vi "ScanBoxA.vi"(11 "YTESTER测试数据":T1 caption="不要修改！") -> (3 "YTESTER结论":T2)   [LabVIEW 2017]
doc: "VIDescription=异步调用一个扫码框！"
uses:
  YtCommon.lvlibp/yt`Step StepBaseInput.ctl
  YtCommon.lvlibp/yt`Step StepResult.ctl
  YtCommon.lvlibp/yt`Step TestData.ctl
  YtCommon.lvlibp/yt`Step System Queue.ctl
  74c99672-6dce-4f91-812f-8692ad59771d.vi
  <vilib>/Utility/error.llb/Clear Errors.vi
  YtCommon.lvlibp/yt`varSystemlib IO Read Variable.vi
  YtCommon.lvlibp
panel:
  in  "YTESTER开放参数":T4={"YTESTER_BaseInput"={"isTest"=FALSE, "isSkip"=FALSE, "StepName"="异步·扫码框A", "OnPass"=enum."Next", "OnFail"=enum."Next", "ReTestNumber"=0.0}, "扫码项目"=["SN："], "扫码项长度"=[], "扫码项文本头匹配"=[], "码不可重复"=TRUE, "窗口位置Left(100)"=100, "窗口位置Top(100)"=100, "满足全部扫码项目后延迟触发测试(s)慎用！"=-1.0, "触发哪些DUTs自动测试？"=""}
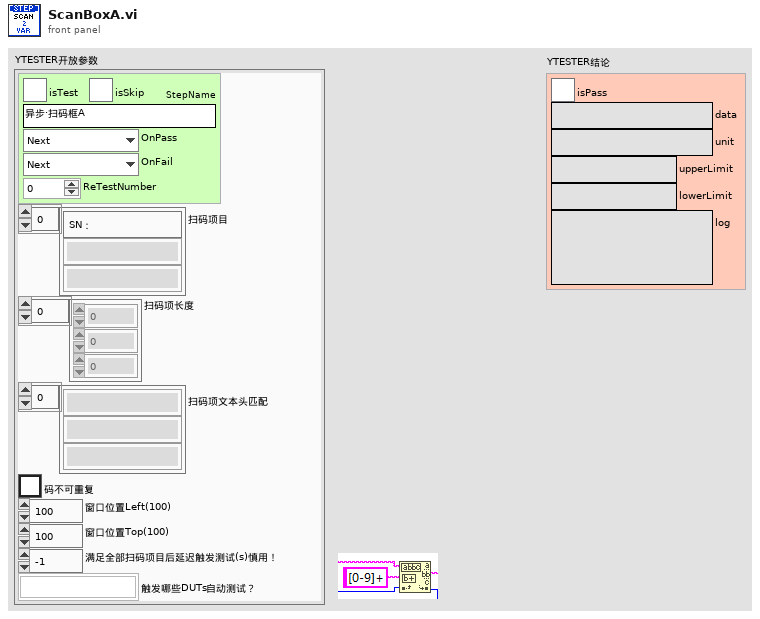
[diagram p1: front panel]
types:
  T1 = typedef "YtCommon.lvlibp/yt`Step TestData.ctl" = cluster{"Socket(From1)":i32, "SN":refnum<notifier>, "StopFlagRef":refnum<notifier>, "YT System Queue":refnum<queue>}
  T2 = typedef "YtCommon.lvlibp/yt`Step StepResult.ctl" = cluster{"isPass":bool, "data":string, "unit":string, "upperLimit":string, "lowerLimit":string, "log":string}
  T3 = typedef "YtCommon.lvlibp/yt`Step StepBaseInput.ctl" = cluster{"isTest":bool, "isSkip":bool, "StepName":string, "OnPass":enum16{"Next", "ToOVER", "Terminate"}, "OnFail":enum16{"Next", "ToOVER", "Terminate"}, "ReTestNumber":dbl}
  T4 = cluster{"YTESTER_BaseInput":T3, "扫码项目":string[], "扫码项长度":u32[], "扫码项文本头匹配":string[], "码不可重复":bool, "窗口位置Left(100)":i16, "窗口位置Top(100)":i16, "满足全部扫码项目后延迟触发测试(s)慎用！":dbl, "触发哪些DUTs自动测试？":string}
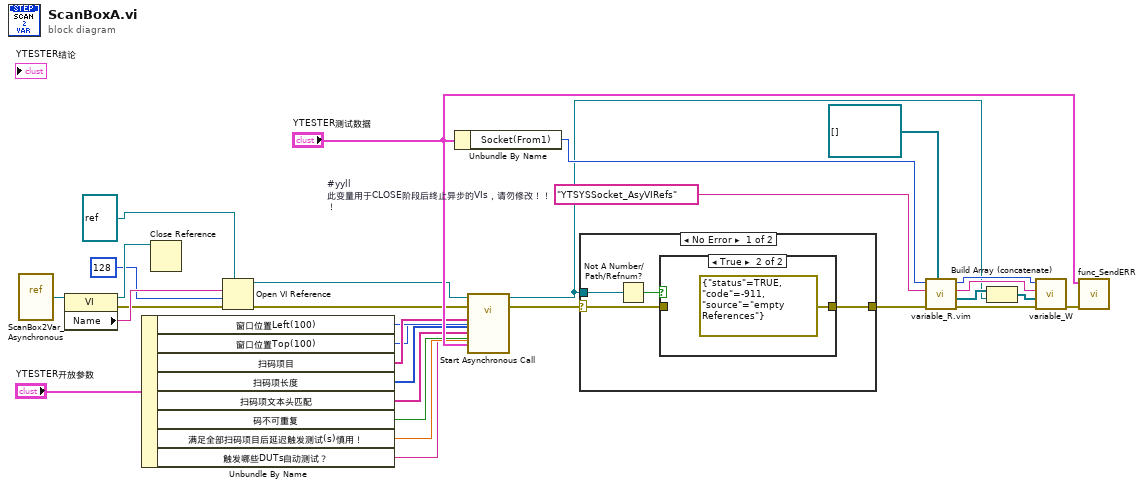
[diagram p0: block diagram]
diagram:
  w7 = "YTSYSSocket_AsyVIRefs"  # #yyll 此变量用于CLOSE阶段后终止异步的VIs，请勿修改！！！
  n1 = vi-ref "ScanBox2Var_Asynchronous.vi"() -> (w30:refnum<vi>)
  n2 = property class="VI"(reference=w30) -> (reference out=w27:refnum<vi>, error out=w28:errorcluster, "Name"=w29:string)  [unwired: 1 in]
  n3 = Unbundle By Name("YTESTER开放参数") -> ("窗口位置Left(100)"=w16:i16, "窗口位置Top(100)"=w15:i16, "扫码项目"=w20:string[], "扫码项长度"=w18:u32[], "扫码项文本头匹配"=w17:string[], "码不可重复"=w19:bool, "满足全部扫码项目后延迟触发测试(s)慎用！"=w5:dbl, "触发哪些DUTs自动测试？"=w1:string)
  n4 = Close Reference(reference=w27) -> ()  [unwired: 1 in, 1 out]
  n5 = Open VI Reference(type specifier VI Refnum (for type only)=refnum<vi> refnum ("VI引用句柄"), vi path=w29, options=128 ("重入简单异步"), error in (no error)=w28) -> (vi reference=w22:refnum<vi>, error out=w24:errorcluster)  [unwired: 2 in]
  n6 = Unbundle By Name("YTESTER测试数据") -> ("Socket(From1)"=w10:i32)
  n7 = call-by-ref "Start Asynchronous Call"(reference=w22, error in=w24, "扫码项目"=w20, "Left(100)"=w16, "Top(100)"=w15, "扫码项长度"=w18, "扫码项文本头匹配"=w17, "码不可重复"=w19, "YTESTER测试数据"="YTESTER测试数据", "满足全部扫码后延迟触发测试（s）"=w5, "触发哪些DUTs自动测试？"=w1) -> (reference out=w2:refnum<vi>, error out=w4:errorcluster)  [unwired: 7 in]
  n8 = case shown="No Error" w4 {
    selector: w4 -> [w32 w37]
    tunnel: w2 -> [w34 _]
    tunnel: [w31 w37] -> w3
    frame No Error {
      n9 = Not A Number/Path/Refnum?(number/path/refnum=w34) -> (NaN/Path/Refnum?=w33:bool)
      n10 = case shown="True" w33 {
        tunnel: [w35 errorcluster {"status"=TRUE, "code"=-911, "source"="empty References"} ("error IO")] -> w31
        tunnel: w32 -> [w35 _]
        frame False {
        }
        frame True {
        }
      }
    }
    frame Error {
    }
  }
  n11 = call "variable_R.vim"("type"=refnum<vi>[] [] ("reference"), "error in"=w3, "待获取变量名称"=w7, "函数池名称"=w10) -> ("error out"=w14:errorcluster, "value"=w12:refnum<vi>[], "待获取变量名out"=w11:string, "函数池名称out"=w9:i32)  [unwired: 3 in, 1 out]
  n12 = Build Array (concatenate)(w12, w2) -> (w13:refnum<vi>[])
  n13 = call "variable_W.vi"("error in (no error)"=w14, "待写入池的输入控件"=w13, "待写入池变量名称"=w11, "函数池名称 in"=w9) -> ("error out"=w6:errorcluster)  [unwired: 5 in, 2 out]
  n14 = call "func_SendERR.vi"("ERR (String\\Errclust)"=w6, "YTESTER测试数据 in"="YTESTER测试数据") -> ()  [unwired: 9 in, 1 out]
